vi "rechts afslaan.vi"(9 "Boolean":bool, 10 "aantal ms rechtdoor":u32, 11 "aantal ms draaien":u32) -> ()   [LabVIEW 2019]
uses:
  <vilib>/myRIO/Common/Instrument Driver Framework/Utilities/typedefs/Analog Scaling Constants.ctl
  <vilib>/myRIO/Common/Instrument Driver Framework/Utilities/typedefs/Analog Scaling Constants List.ctl
  <vilib>/myRIO/Common/Instrument Driver Framework/myRIO v1.0/AO/typedefs/AO Channels Enum.ctl
  <vilib>/myRIO/Common/Instrument Driver Framework/myRIO v1.0/AO/typedefs/AO Channels List.ctl
  <vilib>/myRIO/Common/Instrument Driver Framework/Utilities/typedefs/Generic FPGA Reference.ctl
  <vilib>/myRIO/Common/Instrument Driver Framework/Utilities/typedefs/myRIO v1.0 Reference.ctl
  <vilib>/myRIO/Common/Instrument Driver Framework/Utilities/typedefs/Hardware Version Enum.ctl
  <vilib>/myRIO/Common/Instrument Driver Framework/Utilities/typedefs/myRIO Generic Hardware Reference.ctl
  <vilib>/myRIO/Instrument Drivers/Onboard IO/AO/typedefs/AO Reference.ctl
  <vilib>/myRIO/Instrument Drivers/Onboard IO/AO/AO.lvlib
  <vilib>/myRIO/Instrument Drivers/Onboard IO/AO/vis/Write.vi
  <vilib>/userDefined/High Color/nirio_resource_hc.ctl
  <vilib>/myRIO/Common/Instrument Driver Framework/myRIO v1.0/AO/vis/myRIO v1.1 Open AO.vi
  <vilib>/myRIO/Instrument Drivers/Onboard IO/AO/vis/myRIO AO Open.xnode
  <vilib>/myRIO/Common/Instrument Driver Framework/Utilities/vis/Is FPGA Ref Available.vi
  <vilib>/myRIO/Express VI/Onboard IO/AO/AO Express VI.xnode
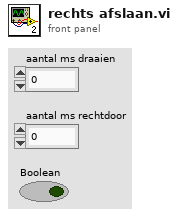
[diagram p1: front panel]
types:
  T1 = typedef "AO.lvlib/AO Reference.ctl" = cluster{"myRIO Reference":T2, "AO Channel List":T6, "AO Scaling Constant List":T8}
  T2 = typedef "myRIO Generic Hardware Reference.ctl" = cluster{"myRIO Model":T3, "myRIO Hardware Reference":T4}
  T3 = typedef "Hardware Version Enum.ctl" = enum16{"Unknown", "myRIO-1900", "myRIO-1950", "roboRIO", "NI ELVIS RIO CM", "ELVIS III"}
  T4 = typedef "myRIO v1.0 Reference.ctl" = cluster{"Generic FPGA Reference":T5, "Allow multiple opens":bool}
  T5 = typedef "Generic FPGA Reference.ctl" = refnum<k20>
  T6 = typedef "AO Channels List.ctl" = T7[]
  T7 = typedef "AO Channels Enum.ctl" = enum16{"Not Connected", "AudioOut/Left", "AudioOut/Right", "C/AO0", "C/AO1", "A/AO0", "A/AO1", "B/AO0", "B/AO1"}
  T8 = typedef "Analog Scaling Constants List.ctl" = T9[]
  T9 = typedef "Analog Scaling Constants.ctl" = cluster{"LSB Weight (Volts)":dbl, "Offset (Volts)":dbl, "Signed?":bool}
  T10 = typedef "nirio_resource_hc.ctl" = tag
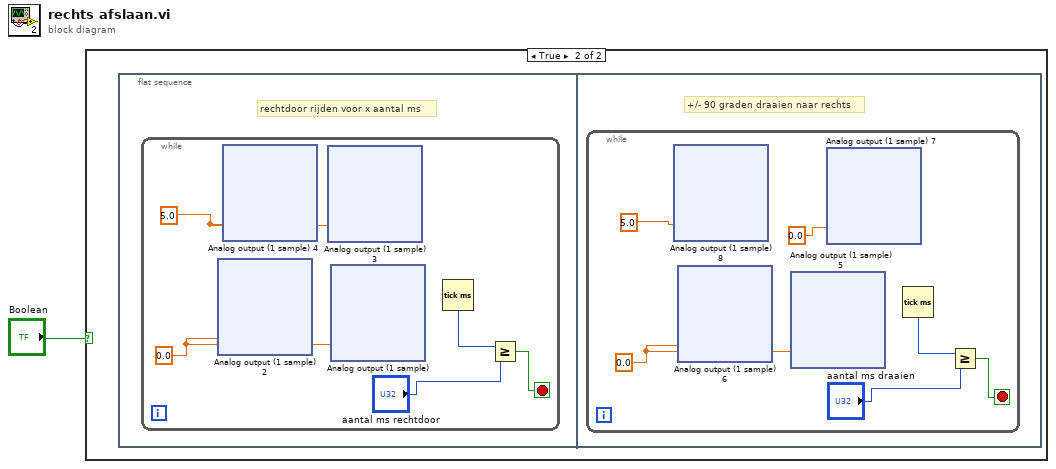
[diagram p0: block diagram]
diagram:
  n1 = case shown="True" "Boolean" {
    frame False {
    }
    frame True {
      n2 = flat-sequence {
        frame #0 {
          # "rechtdoor rijden voor x aantal ms"
          n3 = while {
            stop <- w4 stop-if-true
            w5 = 0.0
            w6 = 5.0
            n4 = xnode "Analog output (1 sample) 2"("A/AO1 (Pin 4)"=w5) -> ()  [unwired: 1 in, 1 out]
            n5 = xnode "Analog output (1 sample) 4"("A/AO0 (Pin 2)"=w6) -> ()  [unwired: 1 in, 1 out]
            n6 = xnode "Analog output (1 sample) 3"("B/AO0 (Pin 2)"=w6) -> ()  [unwired: 1 in, 1 out]
            n7 = xnode "Analog output (1 sample)"("B/AO1 (Pin 4)"=w5) -> ()  [unwired: 1 in, 1 out]
            n8 = Tick Count (ms)() -> (millisecond timer value=w3:u32)
            n9 = Greater Or Equal?(x=w3, y="aantal ms rechtdoor") -> (x >= y?=w4:bool)
          }
        }
        frame #1 {
          # "+/- 90 graden draaien naar rechts"
          n10 = while {
            stop <- w158 stop-if-true
            w159 = 0.0
            n11 = xnode "Analog output (1 sample) 8"("A/AO0 (Pin 2)"=5.0) -> ()  [unwired: 1 in, 1 out]
            n12 = xnode "Analog output (1 sample) 6"("A/AO1 (Pin 4)"=w159) -> ()  [unwired: 1 in, 1 out]
            n13 = xnode "Analog output (1 sample) 5"("B/AO1 (Pin 4)"=w159) -> ()  [unwired: 1 in, 1 out]
            n14 = xnode "Analog output (1 sample) 7"("B/AO0 (Pin 2)"=0.0) -> ()  [unwired: 1 in, 1 out]
            n15 = Tick Count (ms)() -> (millisecond timer value=w157:u32)
            n16 = Greater Or Equal?(x=w157, y="aantal ms draaien") -> (x >= y?=w158:bool)
          }
        }
      }
    }
  }
